vi "Start Trigger Multiple Analogs Channels.vi"(6 "Event types (Edge or Level)":u16(ring) items=["EDGE", "LEVEL"], 8 "error in (no error)":errorcluster, 9 "Complex trigger compare OR or AND":u16(ring) items=["OR", "AND"], 10 "Array of Complex Trigger Consigns":T1[](array[typedef]) {"Channel" items=["A1"=0, "A2"=1, "A3"=2, "A4"=3, "A5"=4, "A6"=5, "A7"=6, "A8"=7, "A9"=8, "A10"=9, "K1"=200, "K2"=201, "K3"=202, "K4"=203, "FA1"=204, "FA2"=205, "FA3"=206, "FA4"=207]; "Assign to S1 or S2 threshold?" items=["S1", "S2"]; "Positive or negative (edge or level)" items=["Positive", "Negative"]}, 11 "VISA resource name":refnum<visa-resource-name>) -> (0 "error out":errorcluster, 3 "VISA resource name out":refnum<visa-resource-name>)   [LabVIEW 2017, in "Sefram DAS220.lvlib"]
doc: "Start on multiple trigger conditions.\nFor example : start record when A3 up to 6V AND/OR A1 down to -4V."
uses:
  <instrlib>/Sefram DAS220/Sefram DAS220.lvlib
  <instrlib>/Sefram DAS220/Public/Configure/Triggers-Alarms/Low-level/Trigger Types/Complex Trigger Consign.ctl
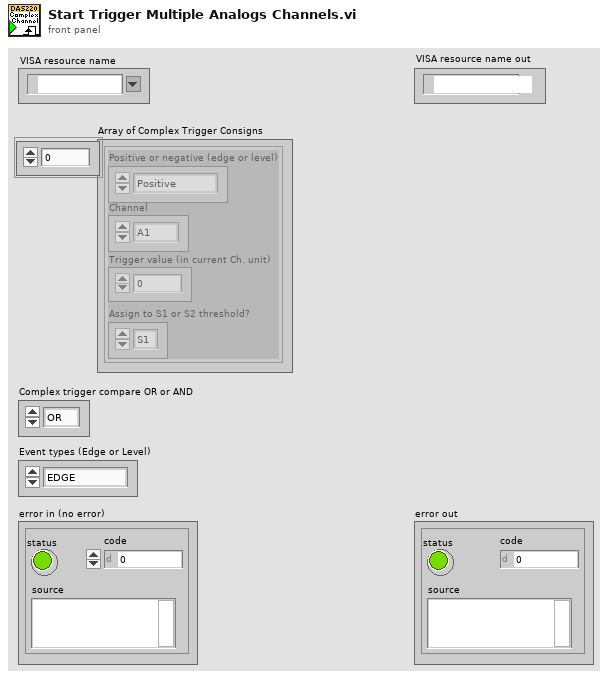
[diagram p1: front panel]
types:
  T1 = typedef "Sefram DAS220.lvlib/Complex Trigger Consign.ctl" = cluster{"Trigger value (in current Ch. unit)":dbl, "Positive or negative (edge or level)":u16, "Assign to S1 or S2 threshold?":u16, "Channel":u16}
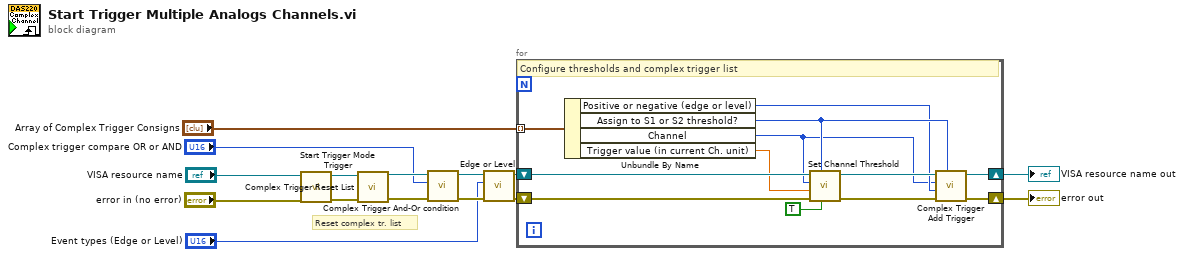
[diagram p0: block diagram]
diagram:
  # "Reset complex tr. list"
  n1 = call <instrlib>:"Start Trigger Mode Trigger.vi"("error in (no error)"="error in (no error)", "VISA resource name"="VISA resource name") -> ("error out"=w8:errorcluster, "VISA resource name out"=w10:refnum<visa-resource-name>)  [unwired: 8 in]
  n2 = call <instrlib>:"Complex Trigger Reset List.vi"("error in (no error)"=w8, "VISA resource name"=w10) -> ("error out"=w14:errorcluster, "VISA resource name out"=w15:refnum<visa-resource-name>)  [unwired: 8 in]
  n3 = call <instrlib>:"Complex Trigger And-Or condition.vi"("error in (no error)"=w14, "Complex trigger compare OR or AND"="Complex trigger compare OR or AND", "VISA resource name"=w15) -> ("error out"=w7:errorcluster, "VISA resource name out"=w5:refnum<visa-resource-name>)  [unwired: 7 in]
  n4 = call <instrlib>:"Edge or Level.vi"("error in (no error)"=w7, "Event types (Edge or Level)"="Event types (Edge or Level)", "VISA resource name"=w5) -> ("error out"=w6:errorcluster, "VISA resource name out"=w4:refnum<visa-resource-name>)  [unwired: 7 in]
  n5 = for {
    tunnel: "Array of Complex Trigger Consigns" -> [w27] mode=indexing
    shift-right: [w20] -> w13
    shift-left: w4 -> [w26]
    shift-right: [w19] -> w12
    shift-left: w6 -> [w25]
    # "Configure thresholds and complex trigger list"
    n6 = Unbundle By Name(w27) -> ("Positive or negative (edge or level)"=w17:u16, "Assign to S1 or S2 threshold?"=w18:u16, "Channel"=w16:u16, "Trigger value (in current Ch. unit)"=w24:dbl)
    n7 = call <instrlib>:"Set Channel Threshold.vi"("Threshold state?"=TRUE ("Threshold On?"), "Threshold S1/S2"=w18, "error in (no error)"=w25, "Threshold value (in actual channel unit)"=w24, "Channel"=w16, "VISA resource name"=w26) -> ("error out"=w22:errorcluster, "VISA resource name out"=w23:refnum<visa-resource-name>)  [unwired: 4 in]
    n8 = call <instrlib>:"Complex Trigger Add Trigger.vi"("Threshold S1/S2"=w18, "error in (no error)"=w22, "Positive or negative (edge or level)"=w17, "Channel"=w16, "VISA resource name"=w23) -> ("error out"=w19:errorcluster, "VISA resource name out"=w20:refnum<visa-resource-name>)  [unwired: 5 in]
  }
  "VISA resource name out" <- w13
  "error out" <- w12
